vi "2019-05-09_shift_register_2.vi"() -> ()   [LabVIEW 2018]
panel:
  out "Sum":i32
  out "Shift Register Data":i32
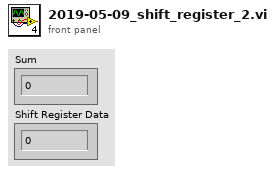
[diagram p1: front panel]
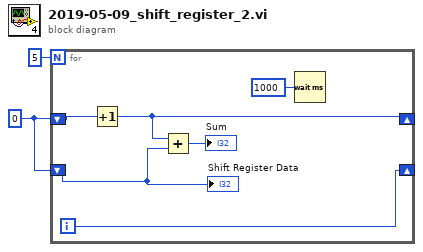
[diagram p0: block diagram]
diagram:
  w1 = 0
  n1 = for {
    N: 5 -> [_]
    shift-right: [w6] -> _
    shift-left: w1 -> [w8]
    shift-right: [w7] -> _
    shift-left: w1 -> [w4]
    i -> [w7]
    n2 = Increment(x=w8) -> (x+1=w6:i32)
    n3 = Add(x=w6, y=w4) -> (x+y=→"Sum":i32)
    n4 = Wait (ms)(milliseconds to wait=u32 1000 ("대기 시간 (ms)")) -> ()  [unwired: 1 out]
    "Shift Register Data" <- w4
  }
